vi "SR430.ProcCases.vi"(0 "i ref in":refnum<vi>, 1 "selector":string, 2 "Data":T1, 3 "call cluster":T2={"Object"="", "Selector"="", "CallType"=enum."synchronous", "Async Object"="", "Async Selector"="", "Data Descriptor"="", "Data"=[], "Error #"=0, "Expire"=0}, 5 "error in (no error)":errorcluster) -> (14 "i ref out":refnum<vi>, 17 "answer cluster":T2={"Object"="", "Selector"="", "CallType"=enum."synchronous", "Async Object"="", "Async Selector"="", "Data Descriptor"="", "Data"=[], "Error #"=0, "Expire"=0}, 19 "error out":errorcluster)   [LabVIEW 2014, in "SR430.lvlib"]
doc: "This method is called by a process from within the default case in the event loop. The methods of a class that are linked to events will be called from THIS method. Add your code here."
uses:
  SR430.lvlib
  CS_Core/CSSystem/CoreDefs/CoreDefs.call_type.ctl
  CS_Core/BaseProcess/BaseProcess.descriptor string definition.ctl
  CS_Core/CSSystem/CoreDefs/CoreDefs.rawDataType.ctl
  CS_Core/CSSystem/CoreLib/CoreLib.string 2 byte array.vi
  CS_Core/CSSystem/CoreLib/CoreLib.byte array 2 int.vi
  CS_Core/CSSystem/CoreLib/CoreLib.int 2 byte array.vi
  CS_Core/CSSystem/CoreLib/CoreLib.byte array 2 short.vi
  CS_Core/CSSystem/CoreLib/CoreLib.byte array 2 double.vi
  CS_Core/CSSystem/CoreLib/CoreLib.double 2 byte array.vi
  CS_Core/CSSystem/CoreLib/CoreLib.short 2 byte array.vi
  CS_Core/CSSystem/CoreLib/CoreLib.lvlib
  CS_Core/BaseProcess/BaseProcess.lvlib
  CS_Core/CSApplicationBaseClasses/DeviceBase/DeviceBase.lvlib
  CS_Core/CSApplicationBaseClasses/MCSBase/MCSBase.lvlib
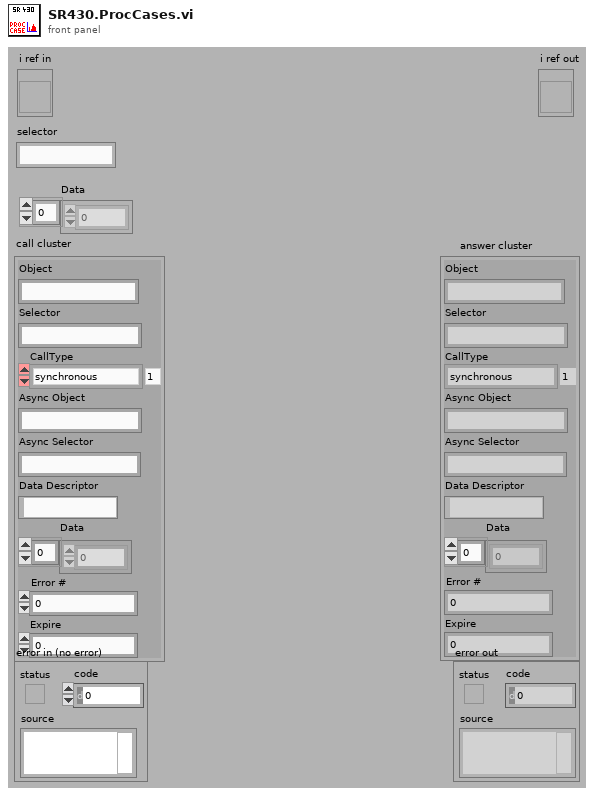
[diagram p1: front panel]
types:
  T1 = typedef "CoreDefs.rawDataType.ctl" = i8[]
  T2 = typedef "CoreDefs.call_type.ctl" = cluster{"Object":string, "Selector":string, "CallType":enum16{"simple", "synchronous", "asynchronous"}, "Async Object":string, "Async Selector":string, "Data Descriptor":T3, "Data":T1, "Error #":i32, "Expire":u32}
  T3 = typedef "BaseProcess.lvlib/BaseProcess.descriptor string definition.ctl" = string
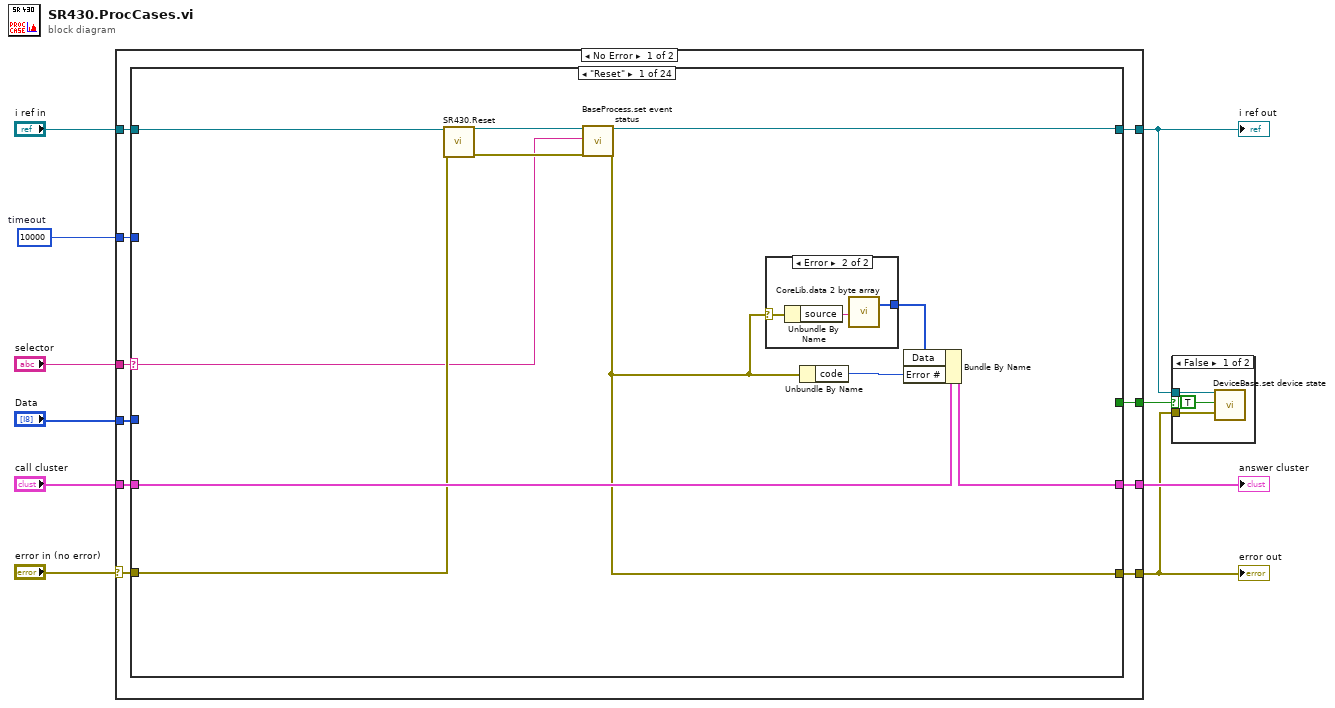
[diagram p0: block diagram]
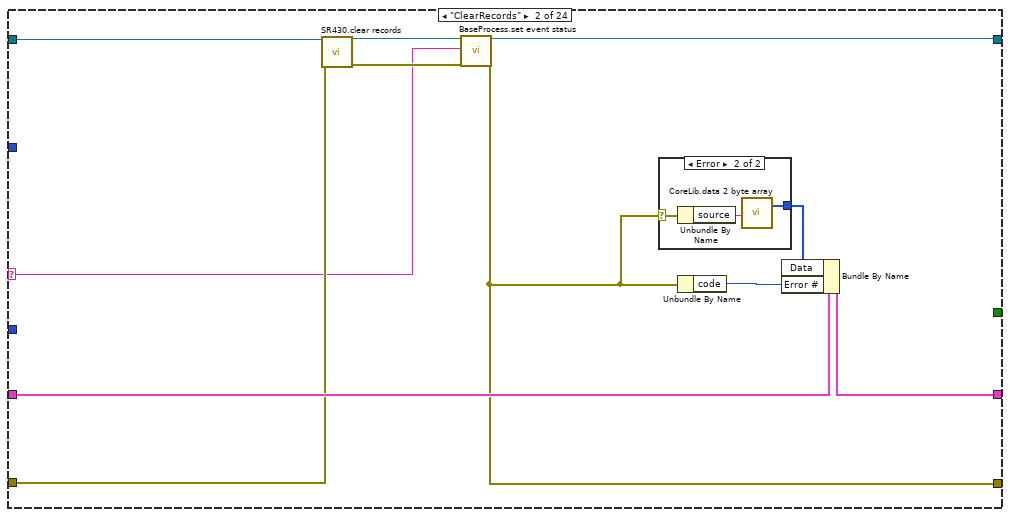
[diagram p3: hidden frame]
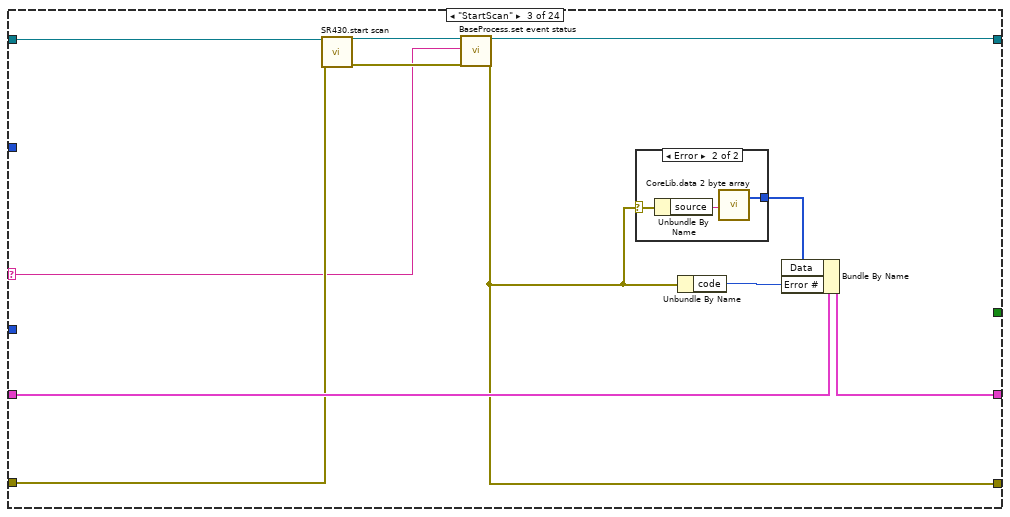
[diagram p5: hidden frame]
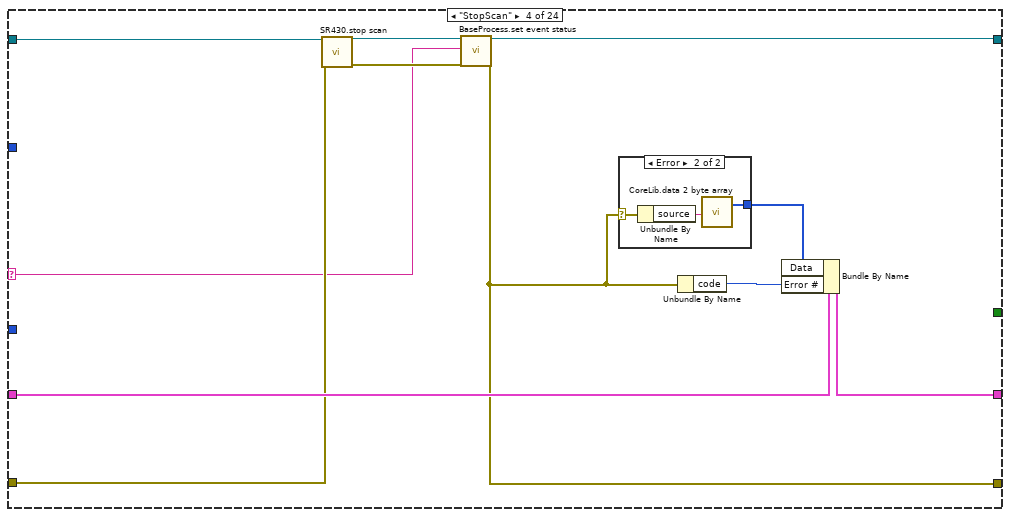
[diagram p7: hidden frame]
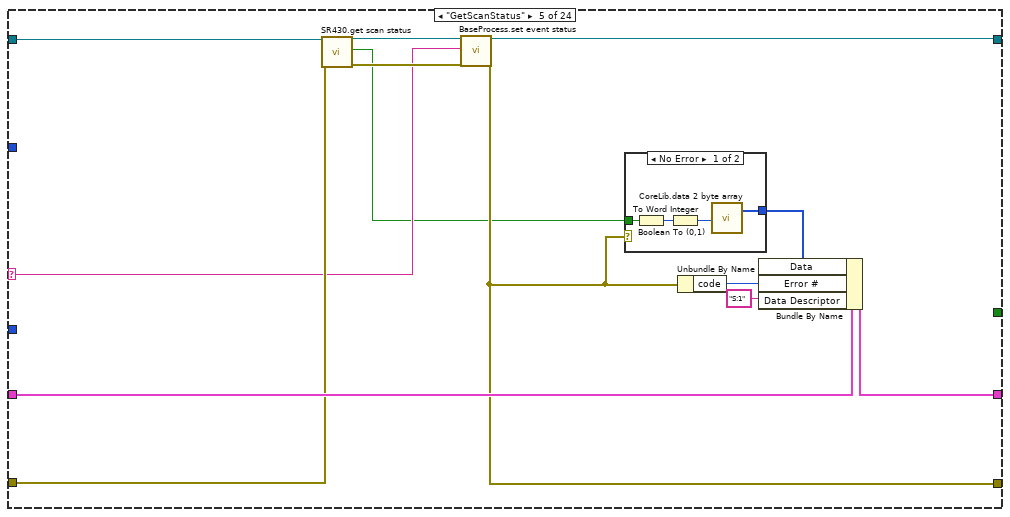
[diagram p9: hidden frame]
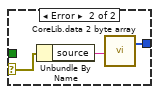
[diagram p10: hidden frame]
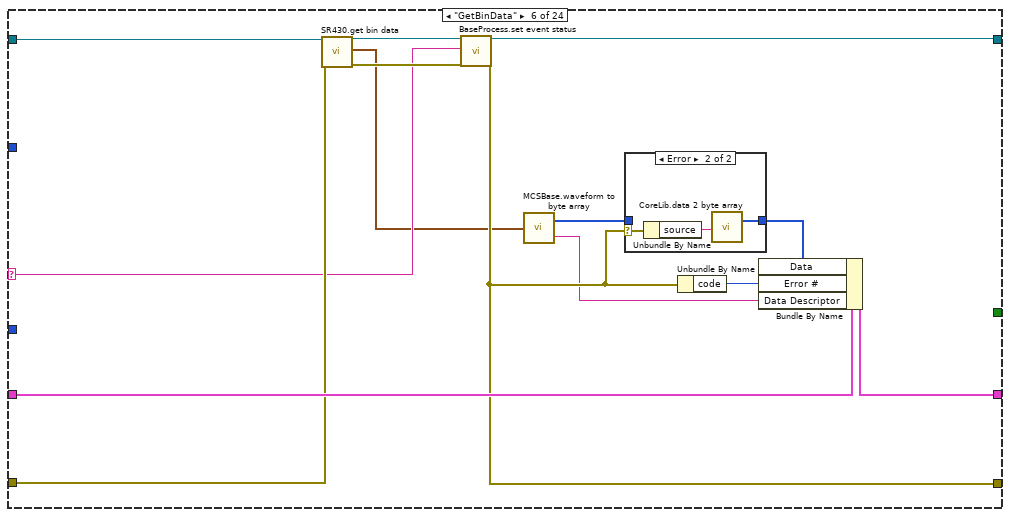
[diagram p11: hidden frame]
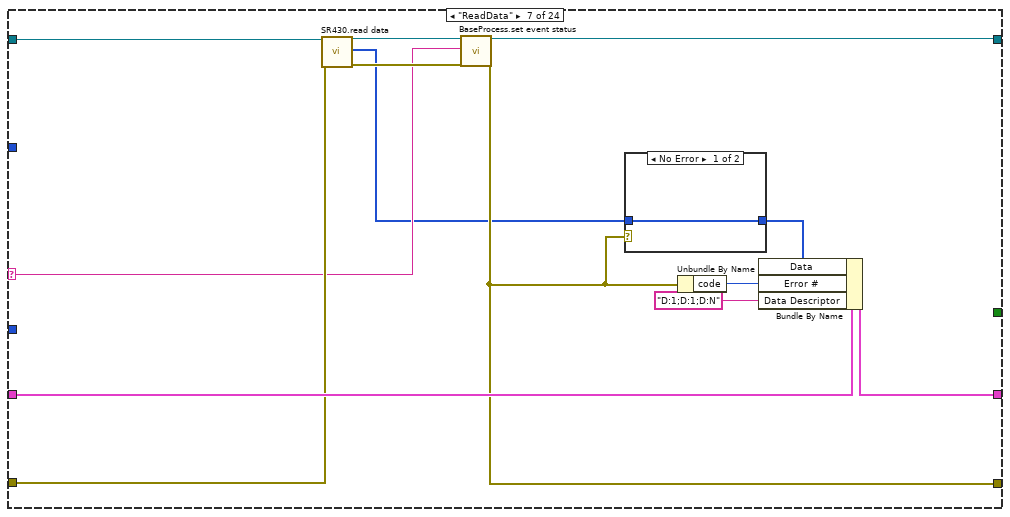
[diagram p13: hidden frame]
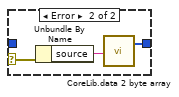
[diagram p14: hidden frame]
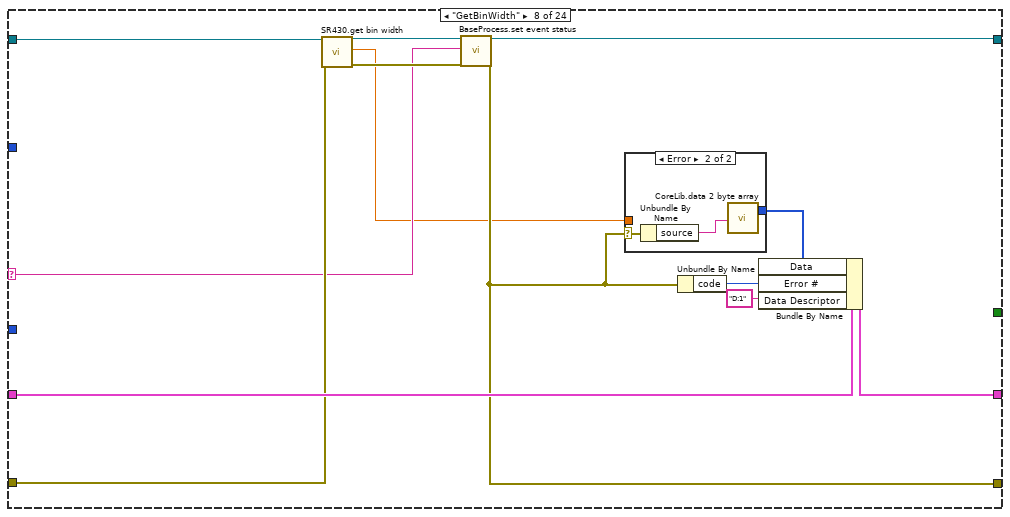
[diagram p15: hidden frame]
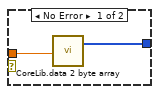
[diagram p16: hidden frame]
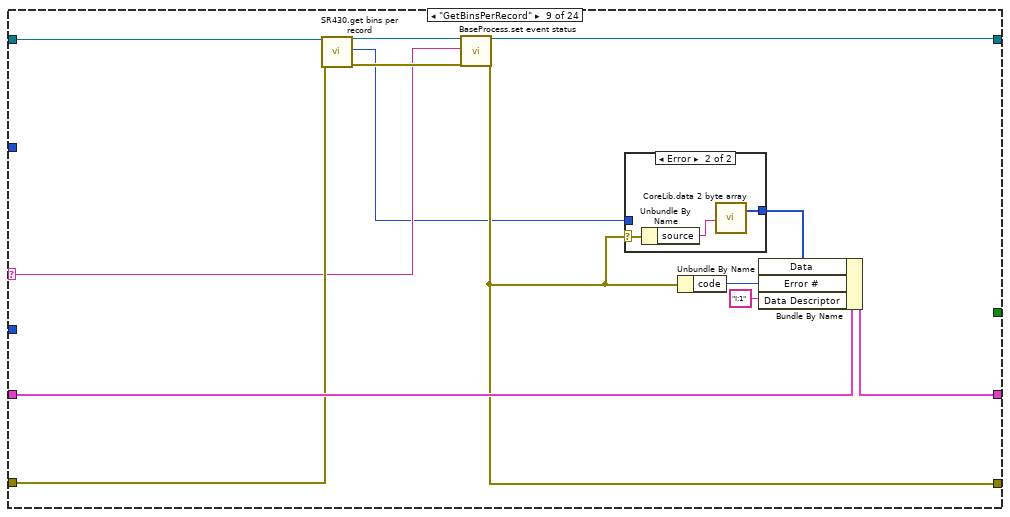
[diagram p17: hidden frame]
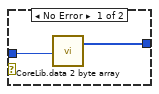
[diagram p18: hidden frame]
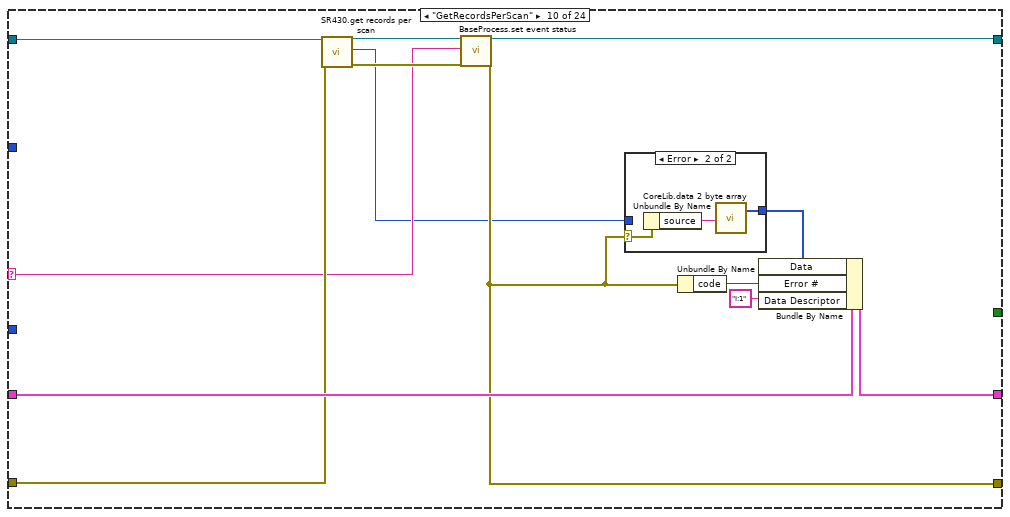
[diagram p19: hidden frame]
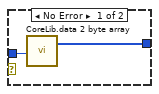
[diagram p20: hidden frame]
diagram:
  w5 = 10000  # timeout
  n1 = case shown="No Error" "error in (no error)" {
    selector: "error in (no error)" -> [w11 w498]
    tunnel: "selector" -> [w20 _]
    tunnel: [w19 w499] -> w9
    tunnel: "Data" -> [w18 _]
    tunnel: "call cluster" -> [w17 w499]
    tunnel: "i ref in" -> [w16 w500]
    tunnel: w5 -> [w15 _]
    tunnel: [w14 w498] -> w4
    tunnel: [w13 w500] -> w3
    tunnel: [w12 _] -> w2
    frame No Error {
      n2 = case shown="\"Reset\"" w20 {
        selector: w20 -> [w21 w37 w51 w65 w79 w100 w117 w134 w152 w170 w188 w206 w225 w242 w274 w301 w327 w354 w381 w414 w440 w466 _ w490]
        tunnel: w18 -> [_ _ _ _ _ _ _ _ _ _ _ _ _ _ _ _ _ _ _ _ _ _ _ w491]
        tunnel: w16 -> [w27 w42 w56 w70 w85 w106 w123 w140 w158 w176 w194 w212 w230 w248 w279 w306 w332 w359 w387 w419 w445 w471 w486 w497]
        tunnel: [w24 w39 w53 w67 w82 w103 w120 w137 w155 w173 w191 w209 w227 w245 w276 w303 w329 w356 w384 w416 w442 w468 w486 w496] -> w13
        tunnel: w17 -> [w31 w45 w59 w73 w89 w110 w127 w144 w162 w180 w198 w216 w224 w241 w273 w300 w326 w353 w380 w413 w439 w465 w488 w492]
        tunnel: [w30 w44 w58 w72 w88 w109 w126 w143 w161 w179 w197 w215 w232 w251 w281 w308 w334 w361 w390 w421 w447 w473 w488 w493] -> w19
        tunnel: w11 -> [w26 w41 w55 w69 w84 w105 w122 w139 w157 w175 w193 w211 w229 w247 w278 w305 w331 w358 w386 w418 w444 w470 w487 w495]
        tunnel: [w22 w36 w50 w64 w80 w101 w118 w135 w153 w171 w189 w207 w223 w243 w268 w296 w322 w349 w382 w408 w434 w460 w487 w494] -> w14
        tunnel: w15 -> [_ _ _ _ _ _ _ _ _ _ _ _ _ _ _ _ _ _ w377 _ _ _ _ _]
        tunnel: [_ _ _ _ _ _ _ _ _ _ _ _ _ _ _ _ _ _ _ _ _ _ _ TRUE] -> w12
        frame "Reset" {
          n3 = call "SR430.Reset.vi"("i ref in"=w27, "error in (no error)"=w26) -> ("i ref out"=w25:refnum<vi>, "error out"=w23:errorcluster)  [unwired: 16 in]
          n4 = call "BaseProcess.set event status.vi"("i ref in"=w25, "EventStatus"=w21, "error in (no error)"=w23) -> ("i ref out"=w24:refnum<vi>, "error out"=w22:errorcluster)  [unwired: 14 in, 1 out]
          n5 = case shown="Error" w22 {
            selector: w22 -> [_ w34]
            tunnel: [_ w32] -> w28
            frame No Error {
            }
            frame Error {
              n6 = Unbundle By Name(w34) -> ("source"=w33:string)
              n7 = call-poly "CoreLib.data 2 byte array.vi"("string"=w33) -> ("byteArray out"=w32:T1)  [unwired: 18 in]
            }
          }
          n8 = Unbundle By Name(w22) -> ("code"=w29:i32)
          n9 = Bundle By Name(cluster=w31, "Data"=w28, "Error #"=w29) -> (w30:T2)
        }
        frame "ClearRecords" {
          n10 = call "SR430.clear records.vi"("i ref in"=w42, "error in (no error)"=w41) -> ("i ref out"=w40:refnum<vi>, "error out"=w38:errorcluster)  [unwired: 16 in]
          n11 = call "BaseProcess.set event status.vi"("i ref in"=w40, "EventStatus"=w37, "error in (no error)"=w38) -> ("i ref out"=w39:refnum<vi>, "error out"=w36:errorcluster)  [unwired: 14 in, 1 out]
          n12 = case shown="Error" w36 {
            selector: w36 -> [_ w48]
            tunnel: [_ w46] -> w35
            frame No Error {
            }
            frame Error {
              n13 = Unbundle By Name(w48) -> ("source"=w47:string)
              n14 = call-poly "CoreLib.data 2 byte array.vi"("string"=w47) -> ("byteArray out"=w46:T1)  [unwired: 18 in]
            }
          }
          n15 = Unbundle By Name(w36) -> ("code"=w43:i32)
          n16 = Bundle By Name(cluster=w45, "Data"=w35, "Error #"=w43) -> (w44:T2)
        }
        frame "StartScan" {
          n17 = call "SR430.start scan.vi"("i ref in"=w56, "error in (no error)"=w55) -> ("i ref out"=w54:refnum<vi>, "error out"=w52:errorcluster)  [unwired: 16 in]
          n18 = call "BaseProcess.set event status.vi"("i ref in"=w54, "EventStatus"=w51, "error in (no error)"=w52) -> ("i ref out"=w53:refnum<vi>, "error out"=w50:errorcluster)  [unwired: 14 in, 1 out]
          n19 = case shown="Error" w50 {
            selector: w50 -> [_ w62]
            tunnel: [_ w60] -> w49
            frame No Error {
            }
            frame Error {
              n20 = Unbundle By Name(w62) -> ("source"=w61:string)
              n21 = call-poly "CoreLib.data 2 byte array.vi"("string"=w61) -> ("byteArray out"=w60:T1)  [unwired: 18 in]
            }
          }
          n22 = Unbundle By Name(w50) -> ("code"=w57:i32)
          n23 = Bundle By Name(cluster=w59, "Data"=w49, "Error #"=w57) -> (w58:T2)
        }
        frame "StopScan" {
          n24 = call "SR430.stop scan.vi"("i ref in"=w70, "error in (no error)"=w69) -> ("i ref out"=w68:refnum<vi>, "error out"=w66:errorcluster)  [unwired: 16 in]
          n25 = call "BaseProcess.set event status.vi"("i ref in"=w68, "EventStatus"=w65, "error in (no error)"=w66) -> ("i ref out"=w67:refnum<vi>, "error out"=w64:errorcluster)  [unwired: 14 in, 1 out]
          n26 = case shown="Error" w64 {
            selector: w64 -> [_ w76]
            tunnel: [_ w74] -> w63
            frame No Error {
            }
            frame Error {
              n27 = Unbundle By Name(w76) -> ("source"=w75:string)
              n28 = call-poly "CoreLib.data 2 byte array.vi"("string"=w75) -> ("byteArray out"=w74:T1)  [unwired: 18 in]
            }
          }
          n29 = Unbundle By Name(w64) -> ("code"=w71:i32)
          n30 = Bundle By Name(cluster=w73, "Data"=w63, "Error #"=w71) -> (w72:T2)
        }
        frame "GetScanStatus" {
          n31 = call "SR430.get scan status.vi"("i ref in"=w85, "error in (no error)"=w84) -> ("i ref out"=w83:refnum<vi>, "scanStatus"=w78:bool, "error out"=w81:errorcluster)  [unwired: 15 in]
          n32 = call "BaseProcess.set event status.vi"("i ref in"=w83, "EventStatus"=w79, "error in (no error)"=w81) -> ("i ref out"=w82:refnum<vi>, "error out"=w80:errorcluster)  [unwired: 14 in, 1 out]
          n33 = case shown="No Error" w80 {
            selector: w80 -> [_ w96]
            tunnel: [w90 w95] -> w86
            tunnel: w78 -> [w93 _]
            frame No Error {
              n34 = Boolean To (0,1)(Boolean=w93) -> (0, 1=w92:i16)
              n35 = To Word Integer(number=w92) -> (16bit integer=w91:i16)
              n36 = call-poly "CoreLib.data 2 byte array.vi"("i16"=w91) -> ("byteArray out"=w90:T1)  [unwired: 18 in]
            }
            frame Error {
              n37 = Unbundle By Name(w96) -> ("source"=w94:string)
              n38 = call-poly "CoreLib.data 2 byte array.vi"("string"=w94) -> ("byteArray out"=w95:T1)  [unwired: 18 in]
            }
          }
          n39 = Unbundle By Name(w80) -> ("code"=w87:i32)
          n40 = Bundle By Name(cluster=w89, "Data"=w86, "Error #"=w87, "Data Descriptor"="S:1") -> (w88:T2)
        }
        frame "GetBinData" {
          n41 = call "SR430.get bin data.vi"("i ref in"=w106, "error in (no error)"=w105) -> ("i ref out"=w104:refnum<vi>, "Output Waveform"=w99:waveform(dbl), "error out"=w102:errorcluster)  [unwired: 15 in]
          n42 = call "BaseProcess.set event status.vi"("i ref in"=w104, "EventStatus"=w100, "error in (no error)"=w102) -> ("i ref out"=w103:refnum<vi>, "error out"=w101:errorcluster)  [unwired: 14 in, 1 out]
          n43 = call "MCSBase.waveform to byte array.vi"("Waveform"=w99) -> ("byteArray out"=w98:T1, "dataDescriptor"=w97:string)
          n44 = case shown="Error" w101 {
            selector: w101 -> [_ w114]
            tunnel: [w111 w113] -> w107
            tunnel: w98 -> [w111 _]
            frame No Error {
            }
            frame Error {
              n45 = Unbundle By Name(w114) -> ("source"=w112:string)
              n46 = call-poly "CoreLib.data 2 byte array.vi"("string"=w112) -> ("byteArray out"=w113:T1)  [unwired: 18 in]
            }
          }
          n47 = Unbundle By Name(w101) -> ("code"=w108:i32)
          n48 = Bundle By Name(cluster=w110, "Data"=w107, "Error #"=w108, "Data Descriptor"=w97) -> (w109:T2)
        }
        frame "ReadData" {
          n49 = call "SR430.read data.vi"("i ref in"=w123, "error in (no error)"=w122) -> ("i ref out"=w121:refnum<vi>, "Output Waveform"=w116:T1, "error out"=w119:errorcluster)  [unwired: 15 in]
          n50 = call "BaseProcess.set event status.vi"("i ref in"=w121, "EventStatus"=w117, "error in (no error)"=w119) -> ("i ref out"=w120:refnum<vi>, "error out"=w118:errorcluster)  [unwired: 14 in, 1 out]
          n51 = case shown="No Error" w118 {
            selector: w118 -> [_ w131]
            tunnel: [w128 w130] -> w124
            tunnel: w116 -> [w128 _]
            frame No Error {
            }
            frame Error {
              n52 = Unbundle By Name(w131) -> ("source"=w129:string)
              n53 = call-poly "CoreLib.data 2 byte array.vi"("string"=w129) -> ("byteArray out"=w130:T1)  [unwired: 18 in]
            }
          }
          n54 = Unbundle By Name(w118) -> ("code"=w125:i32)
          n55 = Bundle By Name(cluster=w127, "Data"=w124, "Error #"=w125, "Data Descriptor"="D:1;D:1;D:N") -> (w126:T2)
        }
        frame "GetBinWidth" {
          n56 = call "SR430.get bin width.vi"("i ref in"=w140, "error in (no error)"=w139) -> ("i ref out"=w138:refnum<vi>, "binWidth [us]"=w133:dbl, "error out"=w136:errorcluster)  [unwired: 15 in]
          n57 = call "BaseProcess.set event status.vi"("i ref in"=w138, "EventStatus"=w134, "error in (no error)"=w136) -> ("i ref out"=w137:refnum<vi>, "error out"=w135:errorcluster)  [unwired: 14 in, 1 out]
          n58 = case shown="Error" w135 {
            selector: w135 -> [_ w149]
            tunnel: [w145 w147] -> w141
            tunnel: w133 -> [w146 _]
            frame No Error {
              n59 = call-poly "CoreLib.data 2 byte array.vi"("f64"=w146) -> ("byteArray out"=w145:T1)  [unwired: 18 in]
            }
            frame Error {
              n60 = Unbundle By Name(w149) -> ("source"=w148:string)
              n61 = call-poly "CoreLib.data 2 byte array.vi"("string"=w148) -> ("byteArray out"=w147:T1)  [unwired: 18 in]
            }
          }
          n62 = Unbundle By Name(w135) -> ("code"=w142:i32)
          n63 = Bundle By Name(cluster=w144, "Data"=w141, "Error #"=w142, "Data Descriptor"="D:1") -> (w143:T2)
        }
        frame "GetBinsPerRecord" {
          n64 = call "SR430.get bins per record.vi"("i ref in"=w158, "error in (no error)"=w157) -> ("i ref out"=w156:refnum<vi>, "bins per record"=w151:i32, "error out"=w154:errorcluster)  [unwired: 15 in]
          n65 = call "BaseProcess.set event status.vi"("i ref in"=w156, "EventStatus"=w152, "error in (no error)"=w154) -> ("i ref out"=w155:refnum<vi>, "error out"=w153:errorcluster)  [unwired: 14 in, 1 out]
          n66 = case shown="Error" w153 {
            selector: w153 -> [_ w167]
            tunnel: [w163 w166] -> w159
            tunnel: w151 -> [w164 _]
            frame No Error {
              n67 = call-poly "CoreLib.data 2 byte array.vi"("i32"=w164) -> ("byteArray out"=w163:T1)  [unwired: 18 in]
            }
            frame Error {
              n68 = Unbundle By Name(w167) -> ("source"=w165:string)
              n69 = call-poly "CoreLib.data 2 byte array.vi"("string"=w165) -> ("byteArray out"=w166:T1)  [unwired: 18 in]
            }
          }
          n70 = Unbundle By Name(w153) -> ("code"=w160:i32)
          n71 = Bundle By Name(cluster=w162, "Data"=w159, "Error #"=w160, "Data Descriptor"="I:1") -> (w161:T2)
        }
        frame "GetRecordsPerScan" {
          n72 = call "SR430.get records per scan.vi"("i ref in"=w176, "error in (no error)"=w175) -> ("i ref out"=w174:refnum<vi>, "recordsPerScan"=w169:i32, "error out"=w172:errorcluster)  [unwired: 15 in]
          n73 = call "BaseProcess.set event status.vi"("i ref in"=w174, "EventStatus"=w170, "error in (no error)"=w172) -> ("i ref out"=w173:refnum<vi>, "error out"=w171:errorcluster)  [unwired: 14 in, 1 out]
          n74 = case shown="Error" w171 {
            selector: w171 -> [_ w185]
            tunnel: [w181 w184] -> w177
            tunnel: w169 -> [w182 _]
            frame No Error {
              n75 = call-poly "CoreLib.data 2 byte array.vi"("i32"=w182) -> ("byteArray out"=w181:T1)  [unwired: 18 in]
            }
            frame Error {
              n76 = Unbundle By Name(w185) -> ("source"=w183:string)
              n77 = call-poly "CoreLib.data 2 byte array.vi"("string"=w183) -> ("byteArray out"=w184:T1)  [unwired: 18 in]
            }
          }
          n78 = Unbundle By Name(w171) -> ("code"=w178:i32)
          n79 = Bundle By Name(cluster=w180, "Data"=w177, "Error #"=w178, "Data Descriptor"="I:1") -> (w179:T2)
        }
        frame "GetTriggerOffset" {
          n80 = call "SR430.get trig offset.vi"("i ref in"=w194, "error in (no error)"=w193) -> ("i ref out"=w192:refnum<vi>, "triggerOffset [us]"=w187:i32, "error out"=w190:errorcluster)  [unwired: 14 in, 1 out]
          n81 = call "BaseProcess.set event status.vi"("i ref in"=w192, "EventStatus"=w188, "error in (no error)"=w190) -> ("i ref out"=w191:refnum<vi>, "error out"=w189:errorcluster)  [unwired: 14 in, 1 out]
          n82 = case shown="Error" w189 {
            selector: w189 -> [_ w203]
            tunnel: [w199 w202] -> w195
            tunnel: w187 -> [w200 _]
            frame No Error {
              n83 = call-poly "CoreLib.data 2 byte array.vi"("i32"=w200) -> ("byteArray out"=w199:T1)  [unwired: 18 in]
            }
            frame Error {
              n84 = Unbundle By Name(w203) -> ("source"=w201:string)
              n85 = call-poly "CoreLib.data 2 byte array.vi"("string"=w201) -> ("byteArray out"=w202:T1)  [unwired: 18 in]
            }
          }
          n86 = Unbundle By Name(w189) -> ("code"=w196:i32)
          n87 = Bundle By Name(cluster=w198, "Data"=w195, "Error #"=w196, "Data Descriptor"="I:1") -> (w197:T2)
        }
        frame "GetTriggerOffset_us" {
          n88 = call "SR430.Get Trigger Offset us.vi"("i ref in"=w212, "error in (no error)"=w211) -> ("i ref out"=w210:refnum<vi>, "triggerOffset [us]"=w205:dbl, "error out"=w208:errorcluster)  [unwired: 11 in]
          n89 = call "BaseProcess.set event status.vi"("i ref in"=w210, "EventStatus"=w206, "error in (no error)"=w208) -> ("i ref out"=w209:refnum<vi>, "error out"=w207:errorcluster)  [unwired: 14 in, 1 out]
          n90 = case shown="Error" w207 {
            selector: w207 -> [_ w221]
            tunnel: [w217 w220] -> w213
            tunnel: w205 -> [w218 _]
            frame No Error {
              n91 = call-poly "CoreLib.data 2 byte array.vi"("f64"=w218) -> ("byteArray out"=w217:T1)  [unwired: 18 in]
            }
            frame Error {
              n92 = Unbundle By Name(w221) -> ("source"=w219:string)
              n93 = call-poly "CoreLib.data 2 byte array.vi"("string"=w219) -> ("byteArray out"=w220:T1)  [unwired: 18 in]
            }
          }
          n94 = Unbundle By Name(w207) -> ("code"=w214:i32)
          n95 = Bundle By Name(cluster=w216, "Data"=w213, "Error #"=w214, "Data Descriptor"="D:1") -> (w215:T2)
        }
        frame "Init" {
          n96 = call "SR430.init.vi"("i ref in"=w230, "error in (no error)"=w229) -> ("i ref out"=w228:refnum<vi>, "error out"=w226:errorcluster)  [unwired: 16 in]
          n97 = call "BaseProcess.set event status.vi"("i ref in"=w228, "EventStatus"=w225, "error in (no error)"=w226) -> ("i ref out"=w227:refnum<vi>, "error out"=w223:errorcluster)  [unwired: 14 in, 1 out]
          n98 = case shown="Error" w223 {
            selector: w223 -> [_ w235]
            tunnel: [_ w233] -> w222
            frame No Error {
            }
            frame Error {
              n99 = Unbundle By Name(w235) -> ("source"=w234:string)
              n100 = call-poly "CoreLib.data 2 byte array.vi"("string"=w234) -> ("byteArray out"=w233:T1)  [unwired: 18 in]
            }
          }
          n101 = Unbundle By Name(w223) -> ("code"=w231:i32)
          n102 = Bundle By Name(cluster=w224, "Data"=w222, "Error #"=w231) -> (w232:T2)
        }
        frame "SetBinWidth" {
          n103 = Unbundle By Name(w241) -> ("Data"=w240:T1)
          n104 = call-poly "CoreLib.byte array 2 data.vi"("byteArray"=w240) -> ("d64"=w238:dbl, "error out"=w237:errorcluster)  [unwired: 16 in, 1 out]
          n105 = case shown="No Error" w237 {
            tunnel: w248 -> [w257 w259]
            tunnel: w247 -> [w256 w261]
            tunnel: [w255 w259] -> w246
            tunnel: [w254 w262] -> w244
            tunnel: w242 -> [_ w260]
            tunnel: w238 -> [w253 _]
            tunnel: [w252 0.0 ("act bin width")] -> w239
            frame No Error {
              n106 = call "SR430.set bin width.vi"("i ref in"=w257, "binWidth [us]"=w253, "error in (no error)"=w256) -> ("i ref out"=w255:refnum<vi>, "actBinWidth [us]"=w252:dbl, "error out"=w254:errorcluster)  [unwired: 14 in]
            }
            frame Error {
              n107 = call "CoreLib.set data type mismatch.vi"("error in (no error)"=w261, "error source"=w260) -> ("error out"=w262:errorcluster)  [unwired: 17 in]
            }
          }
          n108 = call "BaseProcess.set event status.vi"("i ref in"=w246, "EventStatus"=w242, "error in (no error)"=w244) -> ("i ref out"=w245:refnum<vi>, "error out"=w243:errorcluster)  [unwired: 14 in, 1 out]
          n109 = case shown="Error" w243 {
            selector: w243 -> [_ w267]
            tunnel: [w263 w266] -> w249
            tunnel: w239 -> [w264 _]
            frame No Error {
              n110 = call-poly "CoreLib.data 2 byte array.vi"("f64"=w264) -> ("byteArray out"=w263:T1)  [unwired: 18 in]
            }
            frame Error {
              n111 = Unbundle By Name(w267) -> ("source"=w265:string)
              n112 = call-poly "CoreLib.data 2 byte array.vi"("string"=w265) -> ("byteArray out"=w266:T1)  [unwired: 18 in]
            }
          }
          n113 = Unbundle By Name(w243) -> ("code"=w250:i32)
          n114 = Bundle By Name(cluster=w241, "Data"=w249, "Error #"=w250, "Data Descriptor"="D:1") -> (w251:T2)
        }
        frame "SetTriggerLevel" {
          n115 = Unbundle By Name(w273) -> ("Data"=w272:T1)
          n116 = call-poly "CoreLib.byte array 2 data.vi"("byteArray"=w272) -> ("d64"=w271:dbl, "error out"=w270:errorcluster)  [unwired: 16 in, 1 out]
          n117 = case shown="No Error" w270 {
            tunnel: w279 -> [w289 w290]
            tunnel: w278 -> [w288 w292]
            tunnel: [w287 w290] -> w277
            tunnel: [w286 w293] -> w275
            tunnel: w274 -> [_ w291]
            tunnel: w271 -> [w285 _]
            frame No Error {
              n118 = call "SR430.set trigger level.vi"("i ref in"=w289, "triggerLevel [V]"=w285, "error in (no error)"=w288) -> ("i ref out"=w287:refnum<vi>, "error out"=w286:errorcluster)  [unwired: 15 in]
            }
            frame Error {
              n119 = call "CoreLib.set data type mismatch.vi"("error in (no error)"=w292, "error source"=w291) -> ("error out"=w293:errorcluster)  [unwired: 17 in]
            }
          }
          n120 = call "BaseProcess.set event status.vi"("i ref in"=w277, "EventStatus"=w274, "error in (no error)"=w275) -> ("i ref out"=w276:refnum<vi>, "error out"=w268:errorcluster)  [unwired: 14 in, 1 out]
          n121 = case shown="Error" w268 {
            selector: w268 -> [_ w284]
            tunnel: [_ w282] -> w269
            frame No Error {
            }
            frame Error {
              n122 = Unbundle By Name(w284) -> ("source"=w283:string)
              n123 = call-poly "CoreLib.data 2 byte array.vi"("string"=w283) -> ("byteArray out"=w282:T1)  [unwired: 18 in]
            }
          }
          n124 = Unbundle By Name(w268) -> ("code"=w280:i32)
          n125 = Bundle By Name(cluster=w273, "Data"=w269, "Error #"=w280) -> (w281:T2)
        }
        frame "SetTriggerSlope" {
          n126 = Unbundle By Name(w300) -> ("Data"=w299:T1)
          n127 = call-poly "CoreLib.byte array 2 data.vi"("byteArray"=w299) -> ("i16"=w298:i16, "error out"=w297:errorcluster)  [unwired: 16 in, 1 out]
          n128 = Not Equal To 0?(x=w298) -> (x != 0?=w294:bool)
          n129 = case shown="No Error" w297 {
            tunnel: w306 -> [w316 w317]
            tunnel: w305 -> [w315 w319]
            tunnel: [w314 w317] -> w304
            tunnel: [w313 w320] -> w302
            tunnel: w301 -> [_ w318]
            tunnel: w294 -> [w312 _]
            frame No Error {
              n130 = call "SR430.set trigger slope.vi"("i ref in"=w316, "trigger slope"=w312, "error in (no error)"=w315) -> ("i ref out"=w314:refnum<vi>, "error out"=w313:errorcluster)  [unwired: 15 in]
            }
            frame Error {
              n131 = call "CoreLib.set data type mismatch.vi"("error in (no error)"=w319, "error source"=w318) -> ("error out"=w320:errorcluster)  [unwired: 17 in]
            }
          }
          n132 = call "BaseProcess.set event status.vi"("i ref in"=w304, "EventStatus"=w301, "error in (no error)"=w302) -> ("i ref out"=w303:refnum<vi>, "error out"=w296:errorcluster)  [unwired: 14 in, 1 out]
          n133 = case shown="Error" w296 {
            selector: w296 -> [_ w311]
            tunnel: [_ w309] -> w295
            frame No Error {
            }
            frame Error {
              n134 = Unbundle By Name(w311) -> ("source"=w310:string)
              n135 = call-poly "CoreLib.data 2 byte array.vi"("string"=w310) -> ("byteArray out"=w309:T1)  [unwired: 18 in]
            }
          }
          n136 = Unbundle By Name(w296) -> ("code"=w307:i32)
          n137 = Bundle By Name(cluster=w300, "Data"=w295, "Error #"=w307) -> (w308:T2)
        }
        frame "SetDiscLevel" {
          n138 = Unbundle By Name(w326) -> ("Data"=w325:T1)
          n139 = call-poly "CoreLib.byte array 2 data.vi"("byteArray"=w325) -> ("d64"=w324:dbl, "error out"=w323:errorcluster)  [unwired: 16 in, 1 out]
          n140 = case shown="Error" w323 {
            tunnel: w332 -> [w342 w343]
            tunnel: w331 -> [w341 w345]
            tunnel: [w340 w343] -> w330
            tunnel: [w339 w346] -> w328
            tunnel: w327 -> [_ w344]
            tunnel: w324 -> [w338 _]
            frame No Error {
              n141 = call "SR430.set discriminator level.vi"("i ref in"=w342, "discriminatorLevel [V]"=w338, "error in (no error)"=w341) -> ("i ref out"=w340:refnum<vi>, "error out"=w339:errorcluster)  [unwired: 15 in]
            }
            frame Error {
              n142 = call "CoreLib.set data type mismatch.vi"("error in (no error)"=w345, "error source"=w344) -> ("error out"=w346:errorcluster)  [unwired: 17 in]
            }
          }
          n143 = call "BaseProcess.set event status.vi"("i ref in"=w330, "EventStatus"=w327, "error in (no error)"=w328) -> ("i ref out"=w329:refnum<vi>, "error out"=w322:errorcluster)  [unwired: 14 in, 1 out]
          n144 = case shown="Error" w322 {
            selector: w322 -> [_ w337]
            tunnel: [_ w335] -> w321
            frame No Error {
            }
            frame Error {
              n145 = Unbundle By Name(w337) -> ("source"=w336:string)
              n146 = call-poly "CoreLib.data 2 byte array.vi"("string"=w336) -> ("byteArray out"=w335:T1)  [unwired: 18 in]
            }
          }
          n147 = Unbundle By Name(w322) -> ("code"=w333:i32)
          n148 = Bundle By Name(cluster=w326, "Data"=w321, "Error #"=w333) -> (w334:T2)
        }
        frame "SetDiscSlope" {
          n149 = Unbundle By Name(w353) -> ("Data"=w352:T1)
          n150 = call-poly "CoreLib.byte array 2 data.vi"("byteArray"=w352) -> ("i16"=w351:i16, "error out"=w350:errorcluster)  [unwired: 16 in, 1 out]
          n151 = Not Equal To 0?(x=w351) -> (x != 0?=w347:bool)
          n152 = case shown="Error" w350 {
            tunnel: w359 -> [w369 w370]
            tunnel: w358 -> [w368 w372]
            tunnel: [w367 w370] -> w357
            tunnel: [w366 w373] -> w355
            tunnel: w354 -> [_ w371]
            tunnel: w347 -> [w365 _]
            frame No Error {
              n153 = call "SR430.set discriminator slope.vi"("i ref in"=w369, "discriminator slope"=w365, "error in (no error)"=w368) -> ("i ref out"=w367:refnum<vi>, "error out"=w366:errorcluster)  [unwired: 15 in]
            }
            frame Error {
              n154 = call "CoreLib.set data type mismatch.vi"("error in (no error)"=w372, "error source"=w371) -> ("error out"=w373:errorcluster)  [unwired: 17 in]
            }
          }
          n155 = call "BaseProcess.set event status.vi"("i ref in"=w357, "EventStatus"=w354, "error in (no error)"=w355) -> ("i ref out"=w356:refnum<vi>, "error out"=w349:errorcluster)  [unwired: 14 in, 1 out]
          n156 = case shown="Error" w349 {
            selector: w349 -> [_ w364]
            tunnel: [_ w362] -> w348
            frame No Error {
            }
            frame Error {
              n157 = Unbundle By Name(w364) -> ("source"=w363:string)
              n158 = call-poly "CoreLib.data 2 byte array.vi"("string"=w363) -> ("byteArray out"=w362:T1)  [unwired: 18 in]
            }
          }
          n159 = Unbundle By Name(w349) -> ("code"=w360:i32)
          n160 = Bundle By Name(cluster=w353, "Data"=w348, "Error #"=w360) -> (w361:T2)
        }
        frame "SetBinsPerRecord" {
          n161 = Unbundle By Name(w380) -> ("Data"=w379:T1)
          n162 = call-poly "CoreLib.byte array 2 data.vi"("byteArray"=w379) -> ("i32"=w376:i32, "error out"=w375:errorcluster)  [unwired: 16 in, 1 out]
          n163 = case shown="No Error" w375 {
            tunnel: w387 -> [w397 w399]
            tunnel: w386 -> [w396 w401]
            tunnel: [w395 w399] -> w385
            tunnel: [w394 w402] -> w383
            tunnel: w381 -> [_ w400]
            tunnel: w376 -> [w393 _]
            tunnel: [w392 0 ("act bin width")] -> w378
            tunnel: w377 -> [w391 _]
            frame No Error {
              n164 = call "SR430.set bins per record.vi"("i ref in"=w397, "binsPerRecord"=w393, "ms timeout (10000)"=w391, "error in (no error)"=w396) -> ("i ref out"=w395:refnum<vi>, "actBinsPerRecored"=w392:i32, "error out"=w394:errorcluster)  [unwired: 12 in, 1 out]
            }
            frame Error {
              n165 = call "CoreLib.set data type mismatch.vi"("error in (no error)"=w401, "error source"=w400) -> ("error out"=w402:errorcluster)  [unwired: 17 in]
            }
          }
          n166 = call "BaseProcess.set event status.vi"("i ref in"=w385, "EventStatus"=w381, "error in (no error)"=w383) -> ("i ref out"=w384:refnum<vi>, "error out"=w382:errorcluster)  [unwired: 14 in, 1 out]
          n167 = case shown="No Error" w382 {
            selector: w382 -> [_ w407]
            tunnel: [w403 w406] -> w388
            tunnel: w378 -> [w404 _]
            frame No Error {
              n168 = call-poly "CoreLib.data 2 byte array.vi"("i32"=w404) -> ("byteArray out"=w403:T1)  [unwired: 18 in]
            }
            frame Error {
              n169 = Unbundle By Name(w407) -> ("source"=w405:string)
              n170 = call-poly "CoreLib.data 2 byte array.vi"("string"=w405) -> ("byteArray out"=w406:T1)  [unwired: 18 in]
            }
          }
          n171 = Unbundle By Name(w382) -> ("code"=w389:i32)
          n172 = Bundle By Name(cluster=w380, "Data"=w388, "Error #"=w389, "Data Descriptor"="I:1") -> (w390:T2)
        }
        frame "SetRecordsPerScan" {
          n173 = Unbundle By Name(w413) -> ("Data"=w412:T1)
          n174 = call-poly "CoreLib.byte array 2 data.vi"("byteArray"=w412) -> ("i32"=w411:i32, "error out"=w410:errorcluster)  [unwired: 16 in, 1 out]
          n175 = case shown="No Error" w410 {
            tunnel: w419 -> [w429 w430]
            tunnel: w418 -> [w428 w432]
            tunnel: [w427 w430] -> w417
            tunnel: [w426 w433] -> w415
            tunnel: w414 -> [_ w431]
            tunnel: w411 -> [w425 _]
            frame No Error {
              n176 = call "SR430.set records per scan.vi"("i ref in"=w429, "records per scan"=w425, "error in (no error)"=w428) -> ("i ref out"=w427:refnum<vi>, "error out"=w426:errorcluster)  [unwired: 15 in]
            }
            frame Error {
              n177 = call "CoreLib.set data type mismatch.vi"("error in (no error)"=w432, "error source"=w431) -> ("error out"=w433:errorcluster)  [unwired: 17 in]
            }
          }
          n178 = call "BaseProcess.set event status.vi"("i ref in"=w417, "EventStatus"=w414, "error in (no error)"=w415) -> ("i ref out"=w416:refnum<vi>, "error out"=w408:errorcluster)  [unwired: 14 in, 1 out]
          n179 = case shown="Error" w408 {
            selector: w408 -> [_ w424]
            tunnel: [_ w422] -> w409
            frame No Error {
            }
            frame Error {
              n180 = Unbundle By Name(w424) -> ("source"=w423:string)
              n181 = call-poly "CoreLib.data 2 byte array.vi"("string"=w423) -> ("byteArray out"=w422:T1)  [unwired: 18 in]
            }
          }
          n182 = Unbundle By Name(w408) -> ("code"=w420:i32)
          n183 = Bundle By Name(cluster=w413, "Data"=w409, "Error #"=w420) -> (w421:T2)
        }
        frame "SetTriggerOffset" {
          n184 = Unbundle By Name(w439) -> ("Data"=w438:T1)
          n185 = call-poly "CoreLib.byte array 2 data.vi"("byteArray"=w438) -> ("i32"=w437:i32, "error out"=w436:errorcluster)  [unwired: 16 in, 1 out]
          n186 = case shown="No Error" w436 {
            tunnel: w445 -> [w455 w456]
            tunnel: w444 -> [w454 w458]
            tunnel: [w453 w456] -> w443
            tunnel: [w452 w459] -> w441
            tunnel: w440 -> [_ w457]
            tunnel: w437 -> [w451 _]
            frame No Error {
              n187 = call "SR430.set trig offset.vi"("i ref in"=w455, "triggerOffset"=w451, "error in (no error)"=w454) -> ("i ref out"=w453:refnum<vi>, "error out"=w452:errorcluster)  [unwired: 14 in, 1 out]
            }
            frame Error {
              n188 = call "CoreLib.set data type mismatch.vi"("error in (no error)"=w458, "error source"=w457) -> ("error out"=w459:errorcluster)  [unwired: 17 in]
            }
          }
          n189 = call "BaseProcess.set event status.vi"("i ref in"=w443, "EventStatus"=w440, "error in (no error)"=w441) -> ("i ref out"=w442:refnum<vi>, "error out"=w434:errorcluster)  [unwired: 14 in, 1 out]
          n190 = case shown="Error" w434 {
            selector: w434 -> [_ w450]
            tunnel: [_ w448] -> w435
            frame No Error {
            }
            frame Error {
              n191 = Unbundle By Name(w450) -> ("source"=w449:string)
              n192 = call-poly "CoreLib.data 2 byte array.vi"("string"=w449) -> ("byteArray out"=w448:T1)  [unwired: 18 in]
            }
          }
          n193 = Unbundle By Name(w434) -> ("code"=w446:i32)
          n194 = Bundle By Name(cluster=w439, "Data"=w435, "Error #"=w446) -> (w447:T2)
        }
        frame "SetTriggerOffset_us" {
          n195 = Unbundle By Name(w465) -> ("Data"=w464:T1)
          n196 = call-poly "CoreLib.byte array 2 data.vi"("byteArray"=w464) -> ("i32"=w463:i32, "error out"=w462:errorcluster)  [unwired: 16 in, 1 out]
          n197 = case shown="No Error" w462 {
            tunnel: w471 -> [w481 w482]
            tunnel: w470 -> [w480 w484]
            tunnel: [w479 w482] -> w469
            tunnel: [w478 w485] -> w467
            tunnel: w466 -> [_ w483]
            tunnel: w463 -> [w477 _]
            frame No Error {
              n198 = call "SR430.Set Trigger Offset us.vi"("i ref in"=w481, "triggerOffset [us]"=w477, "error in (no error)"=w480) -> ("i ref out"=w479:refnum<vi>, "error out"=w478:errorcluster)  [unwired: 11 in]
            }
            frame Error {
              n199 = call "CoreLib.set data type mismatch.vi"("error in (no error)"=w484, "error source"=w483) -> ("error out"=w485:errorcluster)  [unwired: 17 in]
            }
          }
          n200 = call "BaseProcess.set event status.vi"("i ref in"=w469, "EventStatus"=w466, "error in (no error)"=w467) -> ("i ref out"=w468:refnum<vi>, "error out"=w460:errorcluster)  [unwired: 14 in, 1 out]
          n201 = case shown="Error" w460 {
            selector: w460 -> [_ w476]
            tunnel: [_ w474] -> w461
            frame No Error {
            }
            frame Error {
              n202 = Unbundle By Name(w476) -> ("source"=w475:string)
              n203 = call-poly "CoreLib.data 2 byte array.vi"("string"=w475) -> ("byteArray out"=w474:T1)  [unwired: 18 in]
            }
          }
          n204 = Unbundle By Name(w460) -> ("code"=w472:i32)
          n205 = Bundle By Name(cluster=w465, "Data"=w461, "Error #"=w472) -> (w473:T2)
        }
        frame "SetLebitSpecial" {
          # "For compatibility reasons to the LEBIT MCS = Scope\nThere the specials make sense. To make some sense out of them here,\nwe need to add some code - for instance trigger offset?"
        }
        frame Default {
          n206 = call "DeviceBase.ProcCases.vi"("i ref in"=w497, "selector"=w490, "Data"=w491, "call cluster"=w492, "error in (no error)"=w495) -> ("i ref out"=w496:refnum<vi>, "answer cluster"=w493:T2, "error out"=w494:errorcluster)  [unwired: 12 in]
        }
      }
    }
    frame Error {
    }
  }
  "answer cluster" <- w9
  "i ref out" <- w3
  "error out" <- w4
  n207 = case shown="False" w2 {
    tunnel: w4 -> [w503 _]
    tunnel: w3 -> [w502 _]
    frame False {
      n208 = call "DeviceBase.set device state.vi"("i ref in"=w502, "implicit"=TRUE, "device error"=w503) -> ()  [unwired: 14 in, 3 out]
    }
    frame True {
    }
  }
